vi "LCR_PlotNamer.vi"(4 "Secondary Ref":refnum<vi>, 5 "Y-Axis":T1, 6 "Primary Ref":refnum<vi>, 7 "X-Axis":T1, 11 "Graph Ref In":refnum<vi>) -> ()   [LabVIEW 2021]
uses:
  Plotting-Axis.ctl
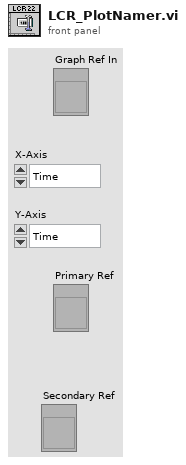
[diagram p1: front panel]
types:
  T1 = typedef "Plotting-Axis.ctl" = enum16{"Time", "Temperature", "MagneticField", "Primary", "Secondary"}
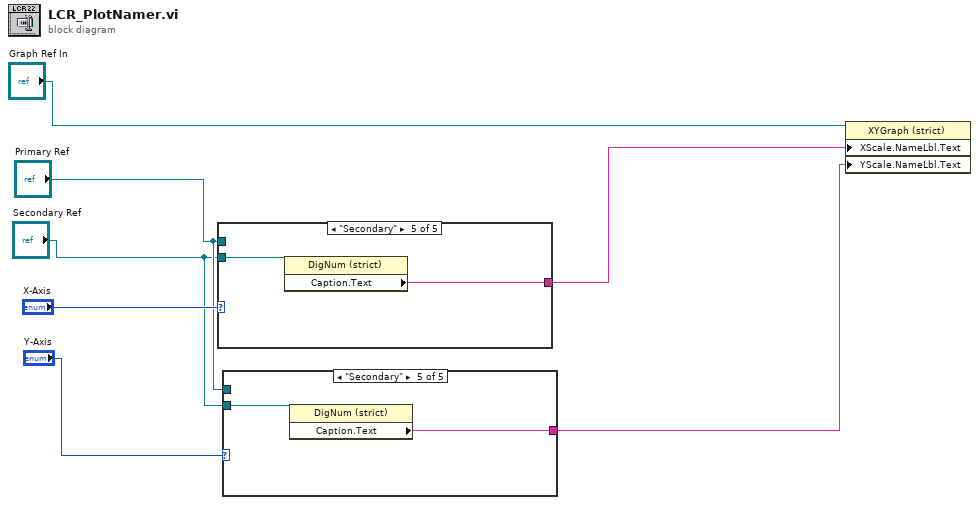
[diagram p0: block diagram]
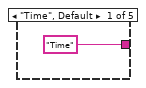
[diagram p2: hidden frame]
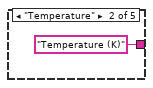
[diagram p3: hidden frame]
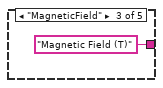
[diagram p4: hidden frame]
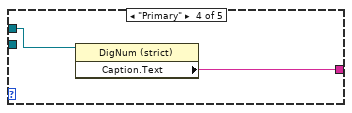
[diagram p5: hidden frame]
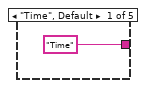
[diagram p6: hidden frame]
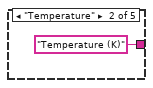
[diagram p7: hidden frame]
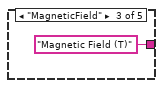
[diagram p8: hidden frame]
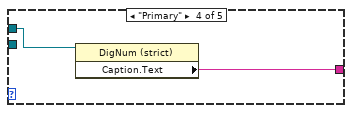
[diagram p9: hidden frame]
diagram:
  n1 = case shown="\"Secondary\"" "X-Axis" {
    tunnel: "Primary Ref" -> [_ _ _ w12 _]
    tunnel: "Secondary Ref" -> [_ _ _ _ w13]
    tunnel: ["Time" "Temperature (K)" ("Caption.Text") "Magnetic Field (T)" ("Caption.Text") w11 w14] -> w2
    frame "Time", Default {
    }
    frame "Temperature" {
    }
    frame "MagneticField" {
    }
    frame "Primary" {
      n2 = property class="DigNum (strict)"(reference=w12) -> ("Caption.Text"=w11:string)  [unwired: 1 in, 2 out]
    }
    frame "Secondary" {
      n3 = property class="DigNum (strict)"(reference=w13) -> ("Caption.Text"=w14:string)  [unwired: 1 in, 2 out]
    }
  }
  n4 = case shown="\"Secondary\"" "Y-Axis" {
    tunnel: "Primary Ref" -> [_ _ _ w19 _]
    tunnel: "Secondary Ref" -> [_ _ _ _ w20]
    tunnel: ["Time" "Temperature (K)" ("Caption.Text") "Magnetic Field (T)" ("Caption.Text") w18 w21] -> w1
    frame "Time", Default {
    }
    frame "Temperature" {
    }
    frame "MagneticField" {
    }
    frame "Primary" {
      n5 = property class="DigNum (strict)"(reference=w19) -> ("Caption.Text"=w18:string)  [unwired: 1 in, 2 out]
    }
    frame "Secondary" {
      n6 = property class="DigNum (strict)"(reference=w20) -> ("Caption.Text"=w21:string)  [unwired: 1 in, 2 out]
    }
  }
  n7 = property class="XYGraph (strict)"(reference="Graph Ref In", "XScale.NameLbl.Text"=w2, "YScale.NameLbl.Text"=w1) -> ()  [unwired: 1 in, 2 out]
